vi "DeviceInfo.vi"() -> ()   [LabVIEW 2020]
panel:
  out "设备信息":T1={"DLL类型"=0, "设备类型"=1, "设备索引"=0, "CAN通道号"=0} {"DLL类型" items=["ControlCAN", "ZLGCAN"]; "设备类型" items=["PCI5121"=1, "PCI9810"=2, "USBCAN1"=3, "USBCAN2"=4, "PCI9820"=5, "PCI5110"=7, "PC104CAN"=11, "CANETUDP"=12, "PCI9840B"=14, "PC104C2"=15, "PCI9820I"=16, "CANETTCP"=17, "PCIE9221"=24, "PCI5010U"=19, "USBCAN_E_U"=20, "USBCAN_2E_U"=21, "PCI5020U"=22, "PCIE9120I"=27, "PCIE9110I"=28, "PCIE9140I"=29]}
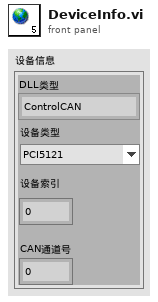
[diagram p1: front panel]
types:
  T1 = cluster{"DLL类型":u32, "设备类型":u32, "设备索引":u32, "CAN通道号":u32}
diagram:
